vi "循环结构的隧道.vi"() -> ()   [LabVIEW 2020]
panel:
  in  "数值 2":i32
  out "字符串":string
  out "字符串":string
  out "循环次数":i32
  out "数值":i32
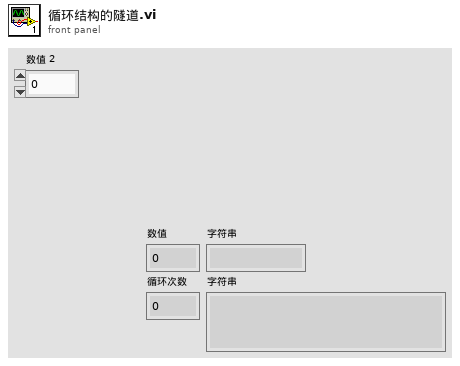
[diagram p1: front panel]
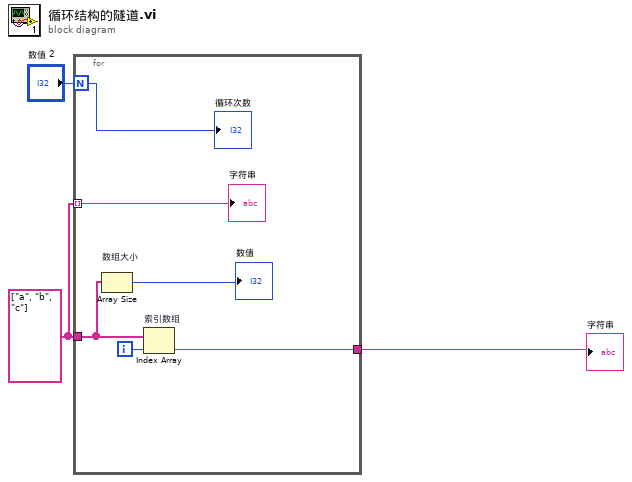
[diagram p0: block diagram]
diagram:
  w3 = string[] ["a", "b", "c"]
  n1 = for {
    N: "数值 2" -> [w8]
    tunnel: w3 -> [w5] mode=indexing
    tunnel: w3 -> [w6]
    tunnel: [w4] -> w2
    i -> [w7]
    n2 = Array Size "数组大小"(array=w6) -> (size(s)=→"数值":i32)
    n3 = Index Array "索引数组"(array=w6, index=w7) -> (element=w4:string)
    "循环次数" <- w8
    "字符串" <- w5
  }
  "字符串" <- w2
